vi "RIO_CheckOperation.vi"(1 "String":string, 2 "Stack in":string[](array[string])) -> (0 "Stack out":string[](array[string]))   [LabVIEW 2012]
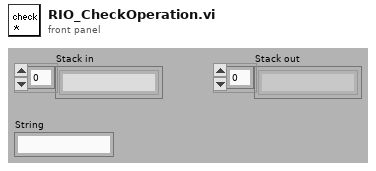
[diagram p1: front panel]
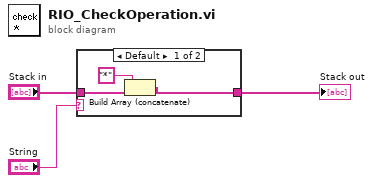
[diagram p0: block diagram]
diagram:
  n1 = case shown="Default" "String" {
    tunnel: "Stack in" -> [w6 w7]
    tunnel: [w5 w7] -> w2
    frame Default {
      n2 = Build Array (concatenate)("*", w6) -> (w5:string[])
    }
    frame "" {
    }
  }
  "Stack out" <- w2
